vi "VFH Speed Selection.vi"(6 "Histogram":dbl[](array[numeric]), 10 "Thresholds":T1, 11 "Max Speed":dbl) -> (3 "Speed":dbl)   [LabVIEW 2016]
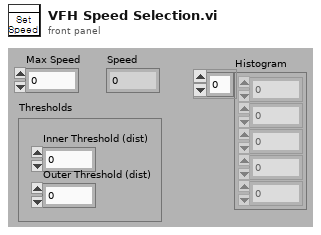
[diagram p1: front panel]
types:
  T1 = cluster{"Inner Threshold (dist)":dbl, "Outer Threshold (dist) ":dbl}
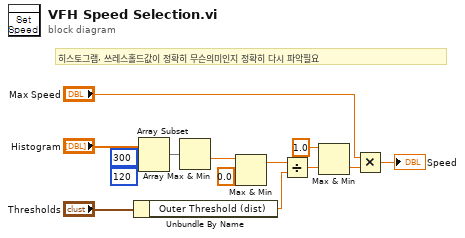
[diagram p0: block diagram]
diagram:
  # "히스토그램, 쓰레스홀드값이 정확히 무슨의미인지 정확히 다시 파악필요"
  n1 = Unbundle By Name("Thresholds") -> ("Outer Threshold (dist)"=w10:dbl)
  n2 = Array Subset(array="Histogram", index=300 ("인덱스"), length=120 ("길이")) -> (w3:dbl[])
  n3 = Array Max & Min(array=w3) -> (min value=w2:dbl)  [unwired: 3 out]
  n4 = Max & Min(x=w2, y=0.0) -> (max(x,y)=w13:dbl)  [unwired: 1 out]
  n5 = Divide(x=w13, y=w10) -> (x/y=w9:dbl)
  n6 = Max & Min(x=1.0, y=w9) -> (min(x,y)=w7:dbl)  [unwired: 1 out]
  n7 = Multiply(x="Max Speed", y=w7) -> (x*y=→"Speed":dbl)
